vi "write_ramp_command.vi"(11 "DAC 1 Ramp Settings":T1={"Ramp Mode"=enum."Fixed", "Ramp Start Value (V)"=0.0, "Ramp Length (Steps)"=1, "Step Width (bins)"=0, "Step Size (V)"=0.0} {"Step Size (V)" min=0.0 max=10.0 step=0.00244 format="%#_4g"; "Step Width (bins)" min=1 max=256; "Ramp Length (Steps)" min=1 max=4096; "Ramp Start Value (V)" min=0.0 max=10.0 step=0.00244}) -> (3 "Command Out":string)   [LabVIEW 2015]
uses:
  Controls/MCS/ramp_control.ctl
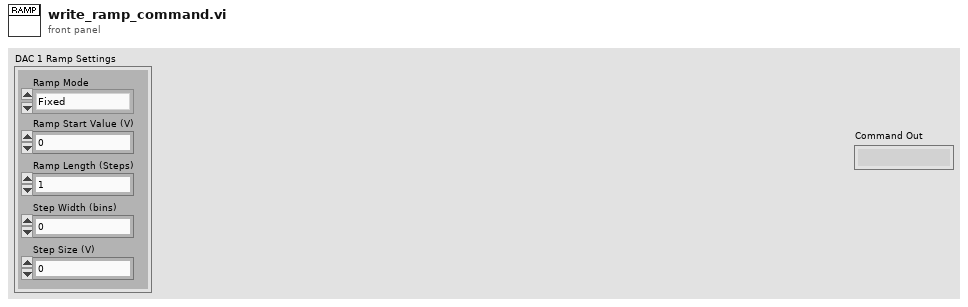
[diagram p1: front panel]
types:
  T1 = typedef "ramp_control.ctl" = cluster{"Ramp Mode":enum16{"Fixed", "Triangle", "Sawtooth"}, "Ramp Start Value (V)":dbl, "Ramp Length (Steps)":i32, "Step Width (bins)":i32, "Step Size (V)":dbl}
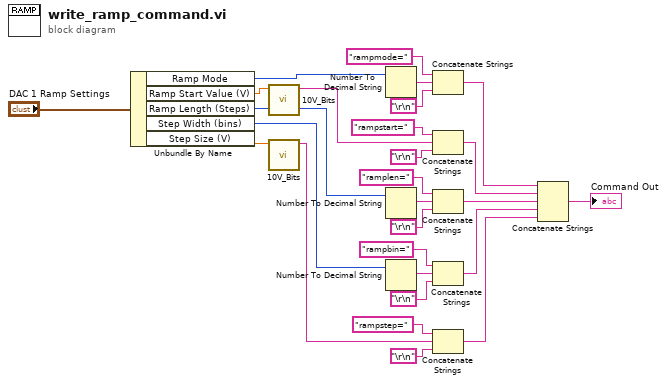
[diagram p0: block diagram]
diagram:
  n1 = Unbundle By Name("DAC 1 Ramp Settings") -> ("Ramp Mode"=w26:enum16{"Fixed", "Triangle", "Sawtooth"}, "Ramp Start Value (V)"=w23:dbl, "Ramp Length (Steps)"=w25:i32, "Step Width (bins)"=w24:i32, "Step Size (V)"=w22:dbl)
  n2 = call "10V_Bits.vi"("Numeric"=w23) -> ("Bits"=w18:string)  [unwired: 10 in]
  n3 = call "10V_Bits.vi"("Numeric"=w22) -> ("Bits"=w9:string)  [unwired: 10 in]
  n4 = Number To Decimal String(number=w26) -> (decimal integer string=w20:string)  [unwired: 1 in]
  n5 = Number To Decimal String(number=w25) -> (decimal integer string=w15:string)  [unwired: 1 in]
  n6 = Number To Decimal String(number=w24) -> (decimal integer string=w12:string)  [unwired: 1 in]
  n7 = Concatenate Strings("rampmode=", w20, "\r\n") -> (w4:string)
  n8 = Concatenate Strings("rampstart=", w18, "\r\n") -> (w5:string)
  n9 = Concatenate Strings("ramplen=", w15, "\r\n") -> (w6:string)
  n10 = Concatenate Strings("rampbin=", w12, "\r\n") -> (w3:string)
  n11 = Concatenate Strings("rampstep=", w9, "\r\n") -> (w2:string)
  n12 = Concatenate Strings(w4, w5, w6, w3, w2) -> (→"Command Out":string)
